vi "Input_1SDI_v00.vi"(11 "Control":T7={"PII In 1"={"Lock"=FALSE, "Hold"=FALSE, "P Gain"=0, "P BS"=-5, "I Gain"=0, "I BS"=-10, "I2 G"=0, "I2 BS"=-26, "Scan Amp"=0, "Scan Off"=0, "Scan FS"=0, "SFS BS"=0, "I Max value"=10000, "I2 Max value"=10000, "Scope.Offset"=0, "Trigger Direction"=enum."either", "Scan-PII thresh"=0}, "PII In 2"={"Lock"=FALSE, "Hold"=FALSE, "P Gain"=0, "P BS"=-10, "I Gain"=0, "I BS"=-10, "I2 G"=0, "I2 BS"=-26, "Scan Amp"=0, "Scan Off"=0, "Scan FS"=0, "SFS BS"=0, "I Max value"=10000, "I2 Max value"=10000, "Scope.Offset"=0, "Trigger Direction"=enum."either", "Scan-PII thresh"=0}, "PII In 3"={"Lock"=FALSE, "Hold"=FALSE, "P Gain"=0, "P BS"=-10, "I Gain"=0, "I BS"=-10, "I2 G"=0, "I2 BS"=-26, "Scan Amp"=0, "Scan Off"=0, "Scan FS"=0, "SFS BS"=0, "I Max value"=10000, "I2 Max value"=10000, "Scope.Offset"=0, "Trigger Direction"=enum."either", "Scan-PII thresh"=0}, "Error scale"={"Pre-Offset"={"Pre-Offset 1"=2, "Pre-Offset 2"=0, "Pre-Offset 3"=0, "Pre-Offset 4"=0, "Pre-Offset 5"=2}, "Post-Offset "={"Offset 1"=0, "Offset 2"=300, "Offset 3"=0, "Offset 4"=0, "Offset 5"=0}, "Gains"={"Gain 1"=0, "Gain 2"=300, "Gain 3"=0, "Gain 4"=0, "Gain 5"=0}, "Bit Shifts"={"Bit Shift 1"=0, "Bit Shift 2"=300, "Bit Shift 3"=0, "Bit Shift 4"=0, "Bit Shift 5"=0}}, "Lock Thresh"={"EPR"=2, "HD A"=0, "HD B"=10}, "Re-Scan Thresh"={"EPR"=2, "HD A"=0, "HD B"=0}, "Theta"={"HD A Sin Theta"=0, "HD A Cos Theta"=0, "HD B Sin Theta"=0, "HD B Cos Theta"=0}, "Safety First"={"lim reset"=FALSE, "no limit"=FALSE, "pos slew rate * dt"=0, "neg slew rate * dt"=-10, "Hold All"=FALSE, "Count(Ticks)"=0}}) -> (3 "Signals":T3={"PII In 1"={"Lock"=FALSE, "Hold"=FALSE, "P Gain"=0, "P BS"=0, "I Gain"=0, "I BS"=-10, "I2 G"=0, "I2 BS"=-26, "Scan Amp"=0, "Scan Off"=0, "Scan FS"=0, "SFS BS"=0, "I Max value"=10000, "I2 Max value"=10000, "Scope.Offset"=0, "Trigger Direction"=enum."either", "Scan-PII thresh"=0}, "PII In 2"={"Lock"=FALSE, "Hold"=FALSE, "P Gain"=0, "P BS"=0, "I Gain"=0, "I BS"=-10, "I2 G"=0, "I2 BS"=-26, "Scan Amp"=0, "Scan Off"=0, "Scan FS"=0, "SFS BS"=0, "I Max value"=10000, "I2 Max value"=10000, "Scope.Offset"=0, "Trigger Direction"=enum."either", "Scan-PII thresh"=0}, "PII In 3"={"Lock"=FALSE, "Hold"=FALSE, "P Gain"=0, "P BS"=0, "I Gain"=0, "I BS"=-10, "I2 G"=0, "I2 BS"=-26, "Scan Amp"=0, "Scan Off"=0, "Scan FS"=0, "SFS BS"=0, "I Max value"=10000, "I2 Max value"=10000, "Scope.Offset"=0, "Trigger Direction"=enum."either", "Scan-PII thresh"=0}, "Lock Thresh"={"EPR"=2, "HD A"=0, "HD B"=0}, "Re-Scan Thresh"={"EPR"=2, "HD A"=0, "HD B"=0}, "Safety First"={"lim reset"=FALSE, "no limit"=FALSE, "pos slew rate * dt"=0, "neg slew rate * dt"=-10, "Hold All"=FALSE, "Count(Ticks)"=4294967286}, "Graph Errors"={"EPR"=2, "HD A"=0, "HD B"=0}}, 7 "HD Errors xp":T1)   [LabVIEW 2011]
doc: "Reads in and scales 8 inputs from the FPGA. For each homodyne lock 2 orthogonal error signals are combined in order to lock the local oscillator to an arbitrary phase."
uses:
  Strict Type Defs/FPGA Inputs 1SDI.ctl
  Strict Type Defs/Error Signals 1SDI.ctl
  Strict Type Defs/Control 1SDI Input.ctl
  Strict Type Defs/PII individual.ctl
  Strict Type Defs/Error Scale 1SDI.ctl
  Strict Type Defs/Lock Thresh 1SDI.ctl
  Strict Type Defs/Theta graph.ctl
  Strict Type Defs/Safety First.ctl
  Strict Type Defs/Signals 1SDI.ctl
  <vilib>/rvi/eio/common/nirviEmuTemplateMethod_errors.vi
  <vilib>/eio/EIONode/EIONode.xnode
panel:
  in  "x p Errors":T1={"HD A x"=0, "HD A p"=1800, "HD B x"=0, "HD B p"=0}
  out "Error Signals":T2={"EPR"=0, "HD A"=1800, "HD B"=0}
  in  "Signals":T3={"PII In 1"={"Lock"=FALSE, "Hold"=FALSE, "P Gain"=0, "P BS"=0, "I Gain"=0, "I BS"=-10, "I2 G"=0, "I2 BS"=-26, "Scan Amp"=0, "Scan Off"=0, "Scan FS"=0, "SFS BS"=0, "I Max value"=10000, "I2 Max value"=10000, "Scope.Offset"=0, "Trigger Direction"=enum."either", "Scan-PII thresh"=0}, "PII In 2"={"Lock"=FALSE, "Hold"=FALSE, "P Gain"=0, "P BS"=0, "I Gain"=0, "I BS"=-10, "I2 G"=0, "I2 BS"=-26, "Scan Amp"=0, "Scan Off"=0, "Scan FS"=0, "SFS BS"=0, "I Max value"=10000, "I2 Max value"=10000, "Scope.Offset"=0, "Trigger Direction"=enum."either", "Scan-PII thresh"=0}, "PII In 3"={"Lock"=FALSE, "Hold"=FALSE, "P Gain"=0, "P BS"=0, "I Gain"=0, "I BS"=-10, "I2 G"=0, "I2 BS"=-26, "Scan Amp"=0, "Scan Off"=0, "Scan FS"=0, "SFS BS"=0, "I Max value"=10000, "I2 Max value"=10000, "Scope.Offset"=0, "Trigger Direction"=enum."either", "Scan-PII thresh"=0}, "Lock Thresh"={"EPR"=2, "HD A"=0, "HD B"=0}, "Re-Scan Thresh"={"EPR"=2, "HD A"=0, "HD B"=0}, "Safety First"={"lim reset"=FALSE, "no limit"=FALSE, "pos slew rate * dt"=0, "neg slew rate * dt"=-10, "Hold All"=FALSE, "Count(Ticks)"=4294967286}, "Graph Errors"={"EPR"=2, "HD A"=0, "HD B"=0}}
  in  "Error Signals":T2
  in  "FPGA Inputs":T10
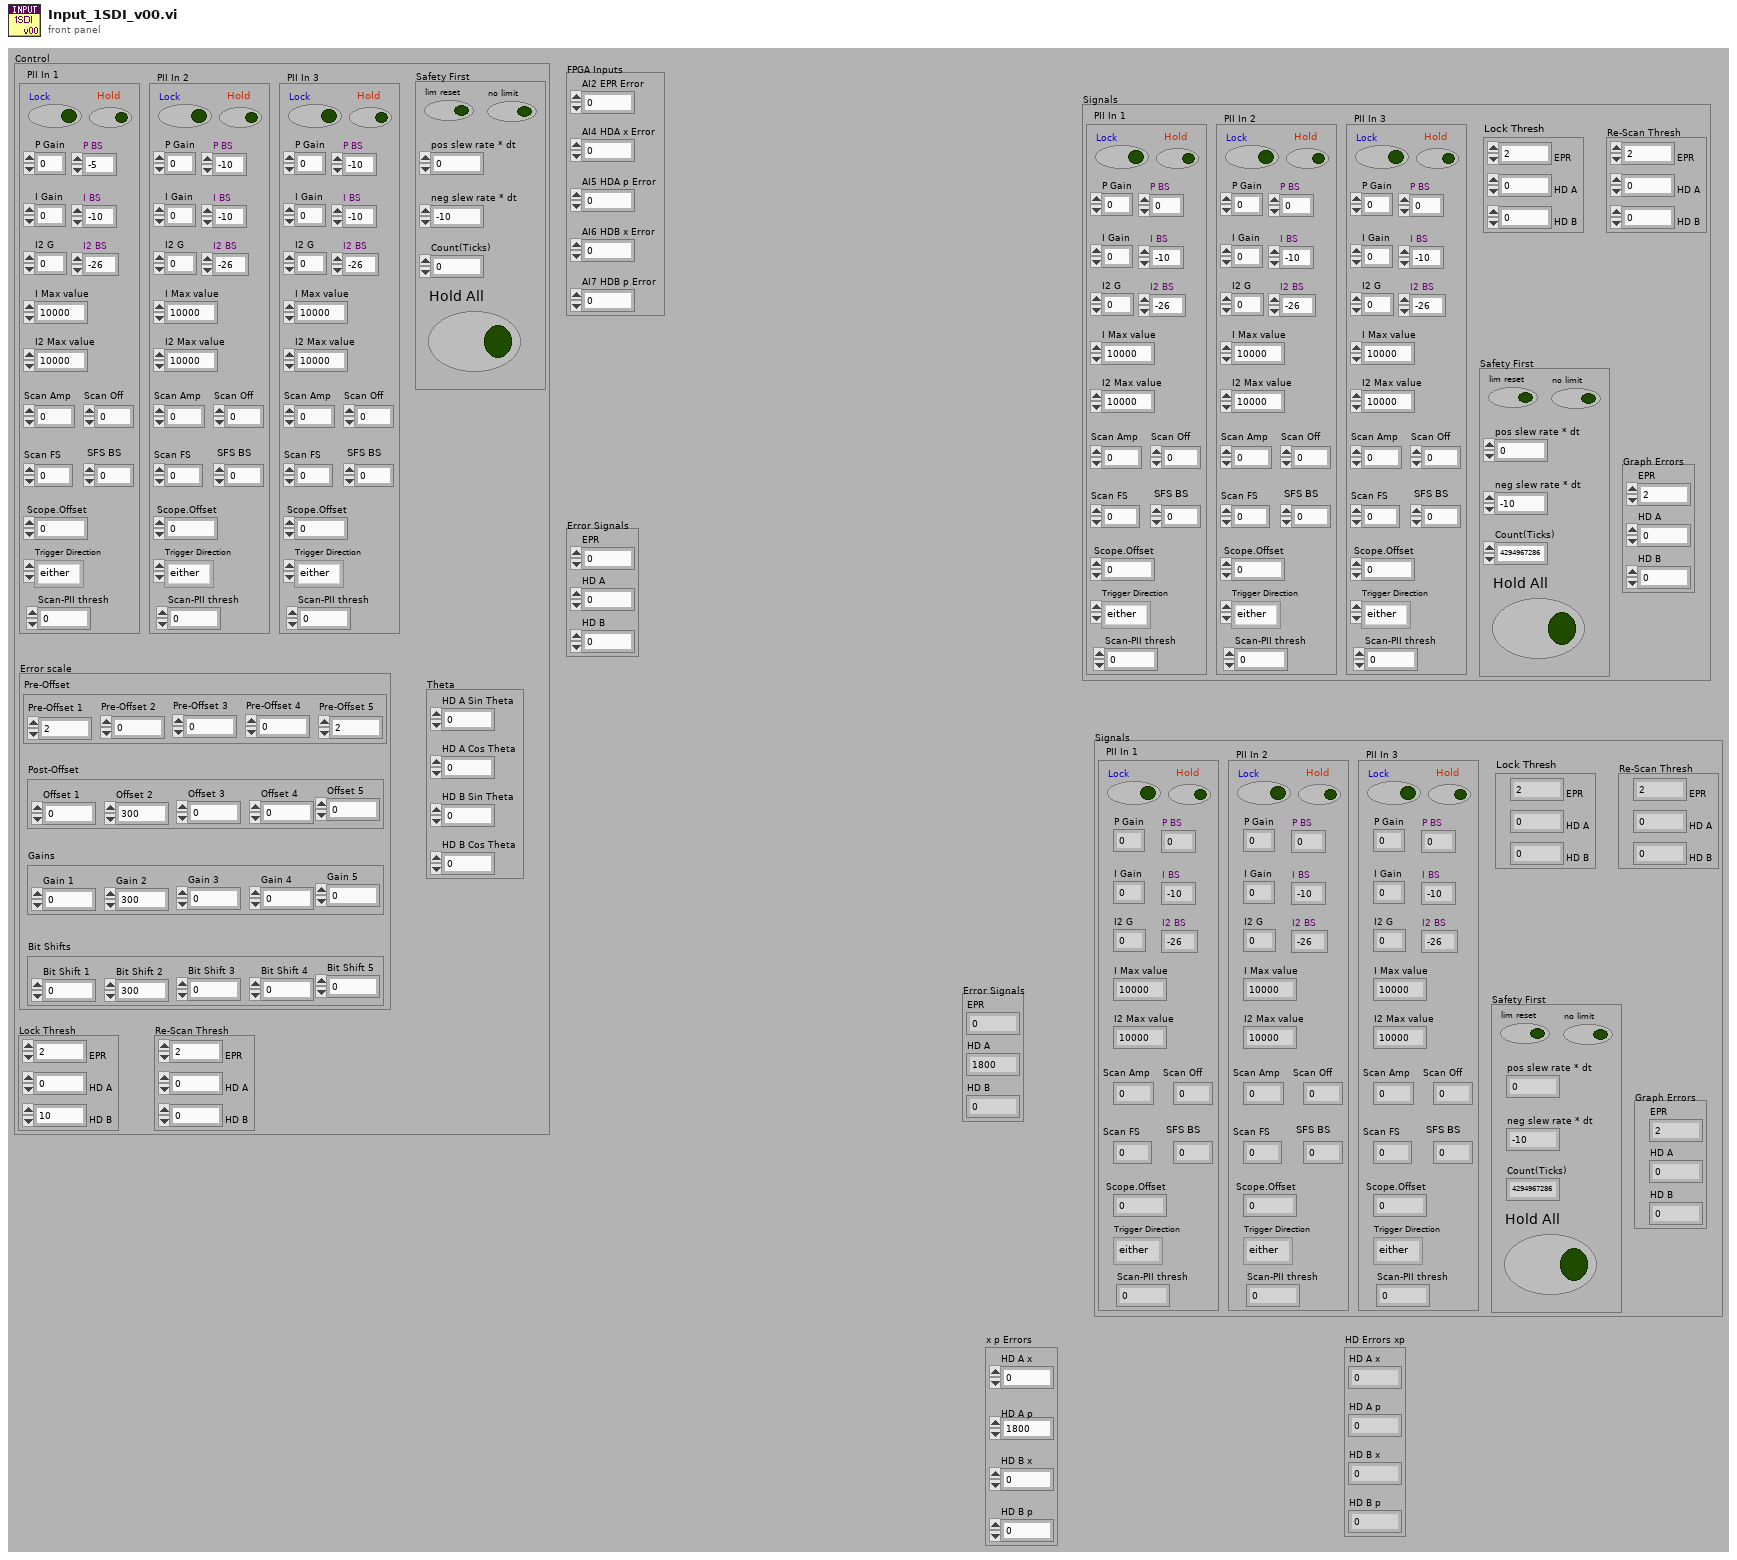
[diagram p1: front panel]
types:
  T1 = cluster{"HD A x":i16, "HD A p":i16, "HD B x":i16, "HD B p":i16}
  T2 = typedef "Error Signals 1SDI.ctl" = cluster{"EPR":i16, "HD A":i16, "HD B":i16}
  T3 = typedef "Signals 1SDI.ctl" = cluster{"PII In 1":T4, "PII In 2":T4, "PII In 3":T4, "Lock Thresh":T5, "Re-Scan Thresh":T5, "Safety First":T6, "Graph Errors":T2}
  T4 = typedef "PII individual.ctl" = cluster{"Lock":bool, "Hold":bool, "P Gain":i32, "P BS":i16, "I Gain":i32, "I BS":i16, "I2 G":i32, "I2 BS":i16, "Scan Amp":i16, "Scan Off":i16, "Scan FS":u16, "SFS BS":i16, "I Max value":i32, "I2 Max value":i32, "Scope.Offset":i16, "Trigger Direction":enum8{"either", "minus-plus", "plus-minus"}, "Scan-PII thresh":i16}
  T5 = typedef "Lock Thresh 1SDI.ctl" = cluster{"EPR":i16, "HD A":i16, "HD B":i16}
  T6 = typedef "Safety First.ctl" = cluster{"lim reset":bool, "no limit":bool, "pos slew rate * dt":i16, "neg slew rate * dt":i16, "Hold All":bool, "Count(Ticks)":u32}
  T7 = typedef "Control 1SDI Input.ctl" = cluster{"PII In 1":T4, "PII In 2":T4, "PII In 3":T4, "Error scale":T8, "Lock Thresh":T5, "Re-Scan Thresh":T5, "Theta":T9, "Safety First":T6}
  T8 = typedef "Error Scale 1SDI.ctl" = cluster{"Pre-Offset":cluster{"Pre-Offset 1":i16, "Pre-Offset 2":i16, "Pre-Offset 3":i16, "Pre-Offset 4":i16, "Pre-Offset 5":i16}, "Post-Offset ":cluster{"Offset 1":i16, "Offset 2":i16, "Offset 3":i16, "Offset 4":i16, "Offset 5":i16}, "Gains":cluster{"Gain 1":i16, "Gain 2":i16, "Gain 3":i16, "Gain 4":i16, "Gain 5":i16}, "Bit Shifts":cluster{"Bit Shift 1":i16, "Bit Shift 2":i16, "Bit Shift 3":i16, "Bit Shift 4":i16, "Bit Shift 5":i16}}
  T9 = typedef "Theta graph.ctl" = cluster{"HD A Sin Theta":i32, "HD A Cos Theta":i32, "HD B Sin Theta":i32, "HD B Cos Theta":i32}
  T10 = typedef "FPGA Inputs 1SDI.ctl" = cluster{"AI2 EPR Error":i16, "AI4 HDA x Error":i16, "AI5 HDA p Error":i16, "AI6 HDB x Error":i16, "AI7 HDB p Error":i16}
  T11 = cluster{"Offset 1":i16, "Offset 2":i16, "Offset 3":i16, "Offset 4":i16, "Offset 5":i16}
  T12 = cluster{"Bit Shift 1":i16, "Bit Shift 2":i16, "Bit Shift 3":i16, "Bit Shift 4":i16, "Bit Shift 5":i16}
  T13 = cluster{"Gain 1":i16, "Gain 2":i16, "Gain 3":i16, "Gain 4":i16, "Gain 5":i16}
  T14 = cluster{"Pre-Offset 1":i16, "Pre-Offset 2":i16, "Pre-Offset 3":i16, "Pre-Offset 4":i16, "Pre-Offset 5":i16}
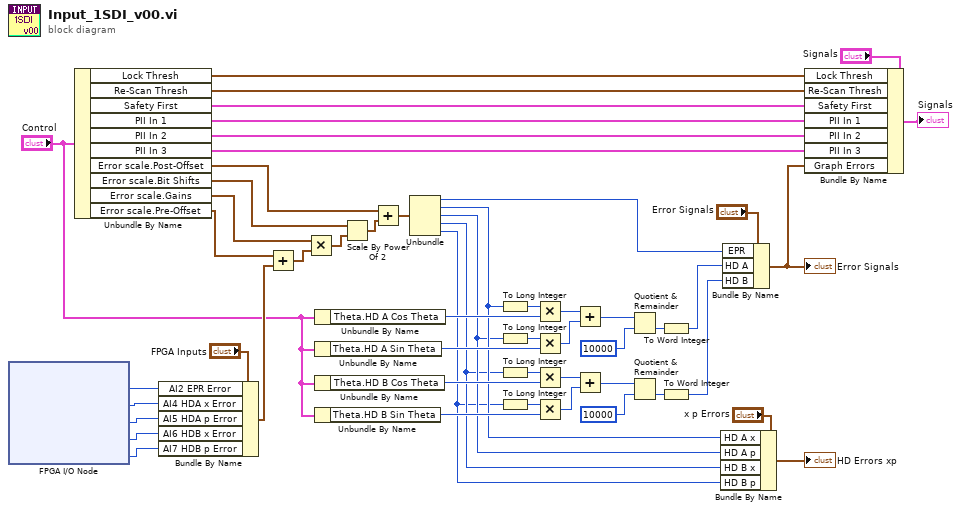
[diagram p0: block diagram]
diagram:
  n1 = xnode "FPGA I/O Node"() -> ("Connector0/AI0"=w10:i16, "Connector0/AI1"=w9:i16, "Connector0/AI2"=w8:i16, "Connector0/AI3"=w7:i16, "Connector0/AI4"=w6:i16)  [unwired: 5 in, 5 out]
  n2 = Unbundle By Name("Control") -> ("Lock Thresh"=w22:T5, "Re-Scan Thresh"=w21:T5, "Safety First"=w23:T6, "PII In 1"=w45:T4, "PII In 2"=w44:T4, "PII In 3"=w43:T4, "Error scale.Post-Offset"=w53:T11, "Error scale.Bit Shifts"=w12:T12, "Error scale.Gains"=w50:T13, "Error scale.Pre-Offset"=w51:T14)
  n3 = Bundle By Name(cluster="FPGA Inputs", "AI2 EPR Error"=w10, "AI4 HDA x Error"=w9, "AI5 HDA p Error"=w8, "AI6 HDB x Error"=w7, "AI7 HDB p Error"=w6) -> (w42:T10)
  n4 = Add(x=w51, y=w42) -> (x+y=w52:T10)
  n5 = Multiply(x=w50, y=w52) -> (x*y=w14:T10)
  n6 = Unbundle By Name("Control") -> ("Theta.HD A Cos Theta"=w39:i32)
  n7 = Unbundle By Name("Control") -> ("Theta.HD A Sin Theta"=w35:i32)
  n8 = Unbundle By Name("Control") -> ("Theta.HD B Cos Theta"=w28:i32)
  n9 = Unbundle By Name("Control") -> ("Theta.HD B Sin Theta"=w32:i32)
  n10 = Scale By Power Of 2(n=w12, x=w14) -> (x*2^n=w13:T10)
  n11 = Add(x=w53, y=w13) -> (x+y=w11:T10)
  n12 = Unbundle(w11) -> ("AI2 EPR Error"=w5:i16, "AI4 HDA x Error"=w4:i16, "AI5 HDA p Error"=w3:i16, "AI6 HDB x Error"=w2:i16, "AI7 HDB p Error"=w1:i16)
  n13 = To Long Integer(number=w4) -> (32bit integer=w40:i32)
  n14 = To Long Integer(number=w3) -> (32bit integer=w36:i32)
  n15 = To Long Integer(number=w2) -> (32bit integer=w27:i32)
  n16 = To Long Integer(number=w1) -> (32bit integer=w31:i32)
  n17 = Multiply(x=w40, y=w39) -> (x*y=w38:i32)
  n18 = Multiply(x=w36, y=w35) -> (x*y=w34:i32)
  n19 = Multiply(x=w27, y=w28) -> (x*y=w29:i32)
  n20 = Multiply(x=w31, y=w32) -> (x*y=w33:i32)
  n21 = Add(x=w38, y=w34) -> (x+y=w37:i32)
  n22 = Add(x=w29, y=w33) -> (x+y=w30:i32)
  n23 = Quotient & Remainder(x=w37, y=10000) -> (floor(x/y)=w18:i32)  [unwired: 1 out]
  n24 = Quotient & Remainder(x=w30, y=10000) -> (floor(x/y)=w20:i32)  [unwired: 1 out]
  n25 = To Word Integer(number=w18) -> (16bit integer=w17:i16)
  n26 = To Word Integer(number=w20) -> (16bit integer=w19:i16)
  n27 = Bundle By Name(cluster="x p Errors", "HD A x"=w4, "HD A p"=w3, "HD B x"=w2, "HD B p"=w1) -> (→"HD Errors xp":T1)
  n28 = Bundle By Name(cluster="Error Signals", "EPR"=w5, "HD A"=w17, "HD B"=w19) -> (w24:T2)
  "Error Signals" <- w24
  n29 = Bundle By Name(cluster="Signals", "Lock Thresh"=w22, "Re-Scan Thresh"=w21, "Safety First"=w23, "PII In 1"=w45, "PII In 2"=w44, "PII In 3"=w43, "Graph Errors"=w24) -> (→"Signals":T3)
